vi "PH_PILS.enable PreAmp.vi"(0 "i ref in":refnum<vi>, 5 "error in":errorcluster) -> (14 "i ref out":refnum<vi>, 19 "error out":errorcluster)   [LabVIEW 2014, in "PH_PILS.lvlib"]
uses:
  PH_PILS.lvlib
  PH_Common/PH_Common.lvlib
  PH_SystemInformation/PH_SystemInformation.lvlib
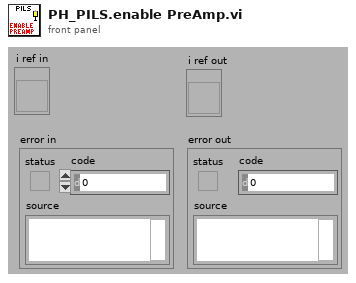
[diagram p1: front panel]
types:
  T1 = typedef "PH_PILS.lvlib/PH_PILS.i attribute.ctl" = cluster{"Boolean":cluster{"GUI Ref":refnum<vi>, "Status":i32}[], "GUI Refs Exp. Shutters":cluster{"1":refnum<vi>, "2":refnum<vi>, "3":refnum<vi>, "4":refnum<vi>}, "Tristate2Run GUI Refs":refnum<vi>[], "EO-Likes":cluster{"GUI Ref":refnum<vi>, "Status":i32}[], "Operation Mode":cluster{"Operation Mode":T2, "GUI":cluster{"Ref State":refnum<vi>, "Ref":refnum<vi>}, "Servicemode":cluster{"Tagname":string, "Status":i32}, "Labormode":cluster{"Tagname":string, "Status":i32}, "Searchmode":cluster{"Tagname":string, "Status":i32}, "Shotmode":cluster{"Tagname":string, "Status":i32}}, "Submode":cluster{"Submode":T3, "GUI":cluster{"Ref State":refnum<vi>, "Ref":refnum<vi>}, "Submode":cluster{"Tagname":string, "Status":i32}}, "Experiment":cluster{"Experiment":enum16{"unknown", "intern", "4 (Z6)", "3", "2", "1"}, "GUI":cluster{"Ref State":refnum<vi>, "Ref":refnum<vi>}, "intern":cluster{"Tagname":string, "Status":i32}, "Exp 4":cluster{"Tagname":string, "Status":i32}, "Exp 3":cluster{"Tagname":string, "Status":i32}, "Exp 2":cluster{"Tagname":string, "Status":i32}, "Exp 1":cluster{"Tagname":string, "Status":i32}}, "TristateNormal":cluster{"GUI Ref":refnum<vi>, "Status":i32}[], "Door Tags":cluster{"GUI Ref":refnum<vi>, "Status":i32}[], "GUIlessTags":cluster{"Name":string, "Status":i32}[], "Beamline GUI Refs":refnum<vi>[], "Special Boolean":cluster{"GUI Ref":refnum<vi>, "Status":i32}[], "Laserpower":cluster{"GUI Ref":refnum<vi>, "Status":i32}[], "Shutter":cluster{"GUI Ref":refnum<vi>, "Status":i32}[], "Tristate EO Like":cluster{"GUI Ref":refnum<vi>, "Status":i32}[], "PP":cluster{"GUI Ref":refnum<vi>, "Status":i32, "Head Ref":refnum<vi>, "Slider Ref":refnum<vi>}[], "Switch Knobs":cluster{"GUI Ref":refnum<vi>, "Status":i32}[], "Latch Knob GUI Refs":refnum<vi>[], "FailureCounter":i32, "Enabled Status":cluster{"Laser":i32, "PreAmp":i32, "MainAmp":i32}, "Mercury":refnum<vi>, "Instance Rods":string, "Logfile":path, "Beckhoff-Instance Internal":string, "Beckhoff-Instance External":string, "Enabling Rights":cluster{"Name":string, "Password":string, "PA?":bool, "MA?":bool, "Exp?":bool}[]}
  T2 = typedef "PH_PILS.lvlib/PH_PILS.Operation Mode.ctl" = enum16{"unknown", "Service", "Labor", "Search", "Shot"}
  T3 = typedef "PH_PILS.lvlib/PH_PILS.Submode.ctl" = enum16{"unknown", "HV-Normal", "HV-Test"}
  T4 = enum16{"Laser", "PreAmp", "MainAmp", "Exp 1", "Exp 2", "Exp 3", "Exp 4"}
  T5 = typedef "PH_SystemInformation.lvlib/PH_SystemInformationEnabling State.ctl" = i32
  T6 = typedef "PH_SystemInformation.lvlib/PH_SystemInformation.i attribute.ctl" = cluster{"Laser Enabling":cluster{"GUI Ref":refnum<vi>, "Enabling State":T5}, "PreAmp Enabling":cluster{"GUI Ref":refnum<vi>, "Enabling State":T5}, "MainAmp Enabling":cluster{"GUI Ref":refnum<vi>, "Enabling State":T5}, "Emergency Off":cluster{"GUI Ref":refnum<vi>, "State":enum16{"no info", "off/false", "Alarm"}}, "Enabling Exp. 1":cluster{"GUI Ref":refnum<vi>, "Enabling State":T5}, "Enabling Exp. 2":cluster{"GUI Ref":refnum<vi>, "Enabling State":T5}, "Enabling Exp. 3":cluster{"GUI Ref":refnum<vi>, "Enabling State":T5}, "Enabling Exp. 4":cluster{"GUI Ref":refnum<vi>, "Enabling State":T5}, "Timing Mode":cluster{"GUI Ref":refnum<vi>, "PHELIX_Timing_Mode":enum32{"10 Hz", "0.5 Hz", "Shot"}}}
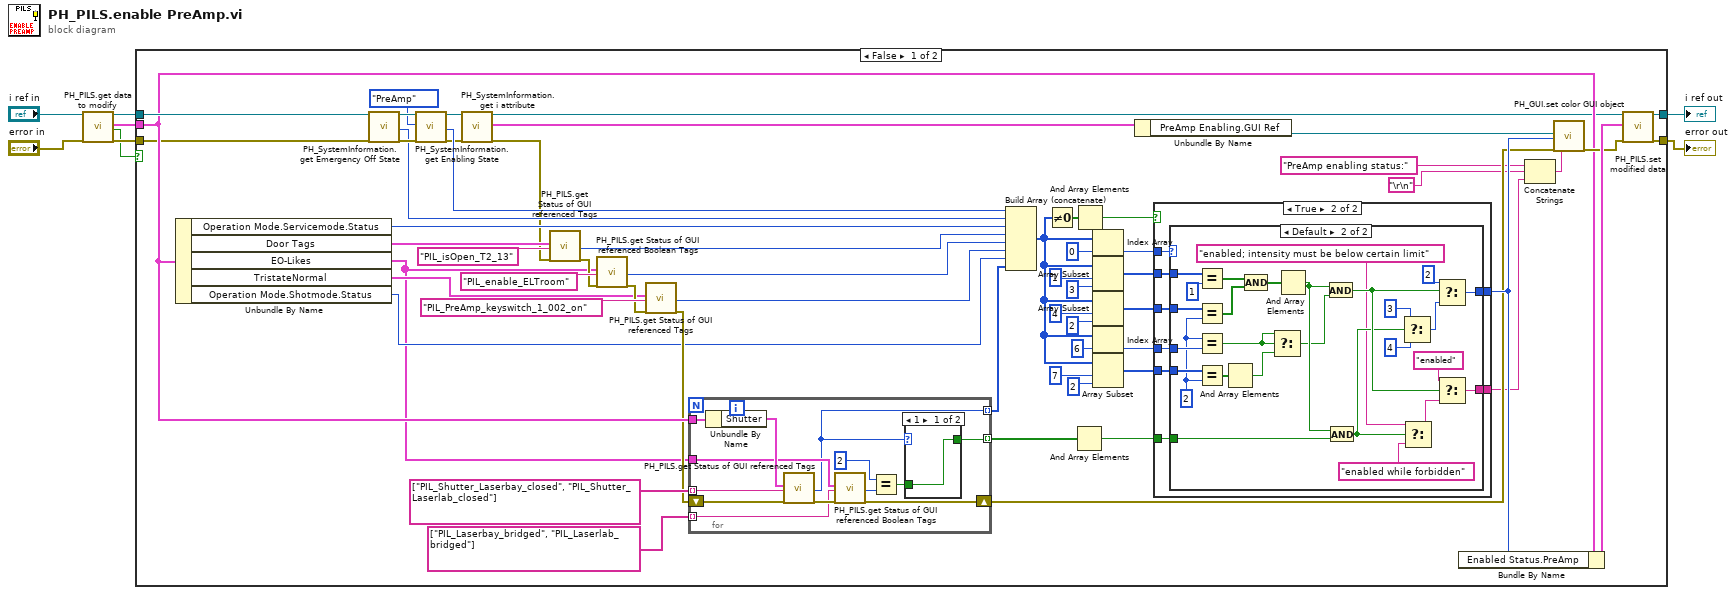
[diagram p0: block diagram]
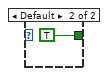
[diagram p2: hidden frame]
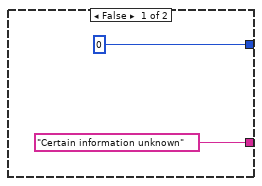
[diagram p3: hidden frame]
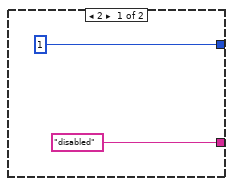
[diagram p4: hidden frame]
diagram:
  n1 = call "PH_PILS.get data to modify.vi"("i ref in"="i ref in", "error in (no error)"="error in") -> ("i ref out"=w4:refnum<vi>, "i attribute"=w5:T1, "timed out"=w3:bool, "error out"=w7:errorcluster)  [unwired: 14 in]
  n2 = case shown="False" w3 {
    tunnel: w7 -> [w21 w122]
    tunnel: w5 -> [w49 _]
    tunnel: [w65 w122] -> w2
    tunnel: w4 -> [w64 w123]
    tunnel: [w63 w123] -> w1
    frame False {
      n3 = Unbundle By Name(w49) -> ("Operation Mode.Servicemode.Status"=w46:i32, "Door Tags"=w58:cluster{"GUI Ref":refnum<vi>, "Status":i32}[], "EO-Likes"=w9:cluster{"GUI Ref":refnum<vi>, "Status":i32}[], "TristateNormal"=w48:cluster{"GUI Ref":refnum<vi>, "Status":i32}[], "Operation Mode.Shotmode.Status"=w13:i32)
      n4 = call "PH_SystemInformation.get Emergency Off State.vi"("i ref in"=w64, "error in (no error)"=w21) -> ("i ref out"=w26:refnum<vi>, "Emergency Off State"=w23:enum16{"no info", "off/false", "Alarm"}, "error out"=w25:errorcluster)  [unwired: 15 in]
      n5 = call "PH_SystemInformation.get Enabling State.vi"("i ref in"=w26, "Wanted State"=T4."PreAmp", "error in (no error)"=w25) -> ("i ref out"=w27:refnum<vi>, "Enabling State"=w24:T5, "error out"=w19:errorcluster)  [unwired: 14 in]
      n6 = call "PH_SystemInformation.get i attribute.vi"("i ref in"=w27, "error in (no error)"=w19) -> ("i ref out"=w30:refnum<vi>, "i attribute"=w29:T6, "error out"=w18:errorcluster)  [unwired: 15 in]
      n7 = call "PH_PILS.get Status of GUI referenced Tags.vi"("Tags"=w58, "Tagname"="PIL_isOpen_T2_13" ("element"), "error in"=w18) -> ("Status"=w59:i32, "error out"=w51:errorcluster)  [unwired: 13 in, 2 out]
      n8 = call "PH_PILS.get Status of GUI referenced Boolean Tags.vi"("Tags"=w9, "Tagname"="PIL_enable_ELTroom", "error in"=w51) -> ("Status"=w53:i32, "error out"=w52:errorcluster)  [unwired: 13 in, 2 out]
      n9 = call "PH_PILS.get Status of GUI referenced Tags.vi"("Tags"=w48, "Tagname"="PIL_PreAmp_keyswitch_1_002_on", "error in"=w52) -> ("Status"=w55:i32, "error out"=w47:errorcluster)  [unwired: 13 in, 2 out]
      n10 = for {
        tunnel: w49 -> [w80]
        tunnel: string[] ["PIL_Shutter_Laserbay_closed", "PIL_Shutter_Laserlab_closed"] -> [w79] mode=indexing
        tunnel: [w70] -> w33 mode=indexing
        shift-right: [w75] -> w20
        shift-left: w47 -> [w78]
        tunnel: string[] ["PIL_Laserbay_bridged", "PIL_Laserlab_bridged"] -> [w74] mode=indexing
        tunnel: [w69] -> w11 mode=indexing
        tunnel: w9 -> [w71]
        n11 = Unbundle By Name(w80) -> ("Shutter"=w77:cluster{"GUI Ref":refnum<vi>, "Status":i32}[])
        n12 = call "PH_PILS.get Status of GUI referenced Tags.vi"("Tags"=w77, "Tagname"=w79, "error in"=w78) -> ("Status"=w70:i32, "error out"=w76:errorcluster)  [unwired: 13 in, 2 out]
        n13 = call "PH_PILS.get Status of GUI referenced Boolean Tags.vi"("Tags"=w71, "Tagname"=w74, "error in"=w76) -> ("Status"=w73:i32, "error out"=w75:errorcluster)  [unwired: 13 in, 2 out]
        n14 = Equal?(x=2 ("y"), y=w73) -> (x = y?=w68:bool)
        n15 = case shown="1" w70 {
          tunnel: [w81 TRUE] -> w69
          tunnel: w68 -> [w81 _]
          frame 1 {
          }
          frame Default {
          }
        }
      }
      n16 = Build Array (concatenate)(w24, w23, w46, w59, w53, w55, w13, w33) -> (w38:T5[])
      n17 = Not Equal To 0?(x=w38) -> (x != 0?=w67:bool[])
      n18 = And Array Elements(Boolean array=w11) -> (logical AND=w10:bool)
      n19 = And Array Elements(Boolean array=w67) -> (logical AND=w66:bool)
      n20 = Index Array(array=w38, index=0) -> (element=w45:T5)
      n21 = Array Subset(array=w38, index=1, length=3) -> (w42:T5[])
      n22 = Array Subset(array=w38, index=4, length=2) -> (w39:T5[])
      n23 = Index Array(array=w38, index=6) -> (element=w32:T5)
      n24 = Array Subset(array=w38, index=7, length=2) -> (w31:T5[])
      n25 = Unbundle By Name(w29) -> ("PreAmp Enabling.GUI Ref"=w28:refnum<vi>)
      n26 = case shown="True" w66 {
        tunnel: [0 ("Status") w92] -> w60
        tunnel: w45 -> [_ w87]
        tunnel: w42 -> [_ w91]
        tunnel: w39 -> [_ w90]
        tunnel: w32 -> [_ w88]
        tunnel: w31 -> [_ w89]
        tunnel: ["Certain information unknown" w86] -> w14
        tunnel: w10 -> [_ w85]
        frame False {
        }
        frame True {
          n27 = case shown="Default" w87 {
            tunnel: [1 ("y") w121] -> w92
            tunnel: w91 -> [_ w119]
            tunnel: w90 -> [_ w118]
            tunnel: w89 -> [_ w117]
            tunnel: w88 -> [_ w114]
            tunnel: ["disabled" w111] -> w86
            tunnel: w85 -> [_ w106]
            frame 2 {
            }
            frame Default {
              w112 = 2 ("y")
              n28 = Equal?(x=w119, y=1) -> (x = y?=w116:bool[])
              n29 = Equal?(x=w118, y=w112) -> (x = y?=w115:bool[])
              n30 = Equal?(x=w112, y=w114) -> (x = y?=w98:bool)
              n31 = Equal?(x=w117, y=w112) -> (x = y?=w97:bool[])
              n32 = And Array Elements(Boolean array=w97) -> (logical AND=w96:bool)
              n33 = Compound Arithmetic op=AND(w116, w115) -> (w109:bool[])
              n34 = Select(t=w98, s=w98, f=w96) -> (s? t:f=w95:bool)
              n35 = And Array Elements(Boolean array=w109) -> (logical AND=w104:bool)
              n36 = And(x=w104, y=w95) -> (x .and. y?=w105:bool)
              n37 = And(x=w104, y=w106) -> (x .and. y?=w102:bool)
              n38 = Select(t=3 ("y"), s=w102, f=4 ("y")) -> (s? t:f=w103:i32)
              n39 = Select(t="enabled; intensity must be below certain limit", s=w102, f="enabled while forbidden") -> (s? t:f=w101:string)
              n40 = Select(t=2 ("y"), s=w105, f=w103) -> (s? t:f=w121:i32)
              n41 = Select(t="enabled", s=w105, f=w101) -> (s? t:f=w111:string)
            }
          }
        }
      }
      n42 = Bundle By Name(cluster=w49, "Enabled Status.PreAmp"=w60) -> (w62:T1)
      n43 = Concatenate Strings("PreAmp enabling status:", "\r\n", w14) -> (w16:string)
      n44 = call "PH_GUI.set color GUI object.vi"("GUI object Ref"=w28, "State"=w60, "error in (no error)"=w20, "Tip Strip (N/A)"=w16) -> ("error out"=w61:errorcluster)  [unwired: 15 in]
      n45 = call "PH_PILS.set modified data.vi"("i ref in"=w30, "i attribute"=w62, "error in (no error)"=w61) -> ("i ref out"=w63:refnum<vi>, "error out"=w65:errorcluster)  [unwired: 15 in]
    }
    frame True {
    }
  }
  "i ref out" <- w1
  "error out" <- w2
